vi "PositionSegments.vi"() -> ()   [LabVIEW 2015]
uses:
  3D Point.ctl
  3D Scene.lvclass
panel:
  in  "Position":T1
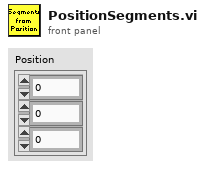
[diagram p1: front panel]
types:
  T1 = typedef "3D Scene.lvclass/3D Point.ctl" = cluster{"X":sgl, "Y":sgl, "Z":sgl}
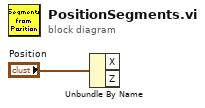
[diagram p0: block diagram]
diagram:
  n1 = Unbundle By Name("Position") -> ()  [unwired: 2 out]
